vi "Serial Transmitter.vi"(9 "Robot":T1={"id"=0, "function"=enum."Attacker", "x"=0.0, "y"=0.0, "orientation"=0.0, "v_tangent"=0.0, "v_normal"=0.0, "v_ang"=0.0, "kick_x"=0.0, "kick_z"=0.0, "dribble"=FALSE, "Timestamp"=timestamp(0 s since 1904-01-01), "estimatives"={"est_v_tangent"=0.0, "est_v_normal"=0.0, "est_vx"=0.0, "est_vy"=0.0, "Pos Robot Est"=[]}, "dest_x_kick"=0.0, "dest_y_kick"=0.0, "Gap Coord"=[], "States"=enum."GoToTangent", "Path "=[], "Path  Smooth"=[], "Dest"=[], "vx_desired"=0.0, "vy_desired"=0.0, "slowBehavior"=FALSE, "VSSStates"=enum."Pass"}, 10 "Porta:":refnum<visa-resource-name>) -> (0 "error out":errorcluster)   [LabVIEW 2023]
uses:
  Vision_class/Old vision/Controls/AI Robot.ctl
  Vision_class/Old vision/Controls/Functions Enum.ctl
  Vision_class/Old vision/Controls/AttackerStates.ctl
  Vision_class/Old vision/Controls/PathDests.ctl
  Vision_class/Old vision/Controls/PathDest.ctl
  Game_class/Navigation/VSSNavigation/VSSAttackerStates.ctl
  <vilib>/Instr/_visa.llb/VISA Configure Serial Port (Instr).vi
panel:
  out "Array":u8[](array[numeric]) format="%02x"
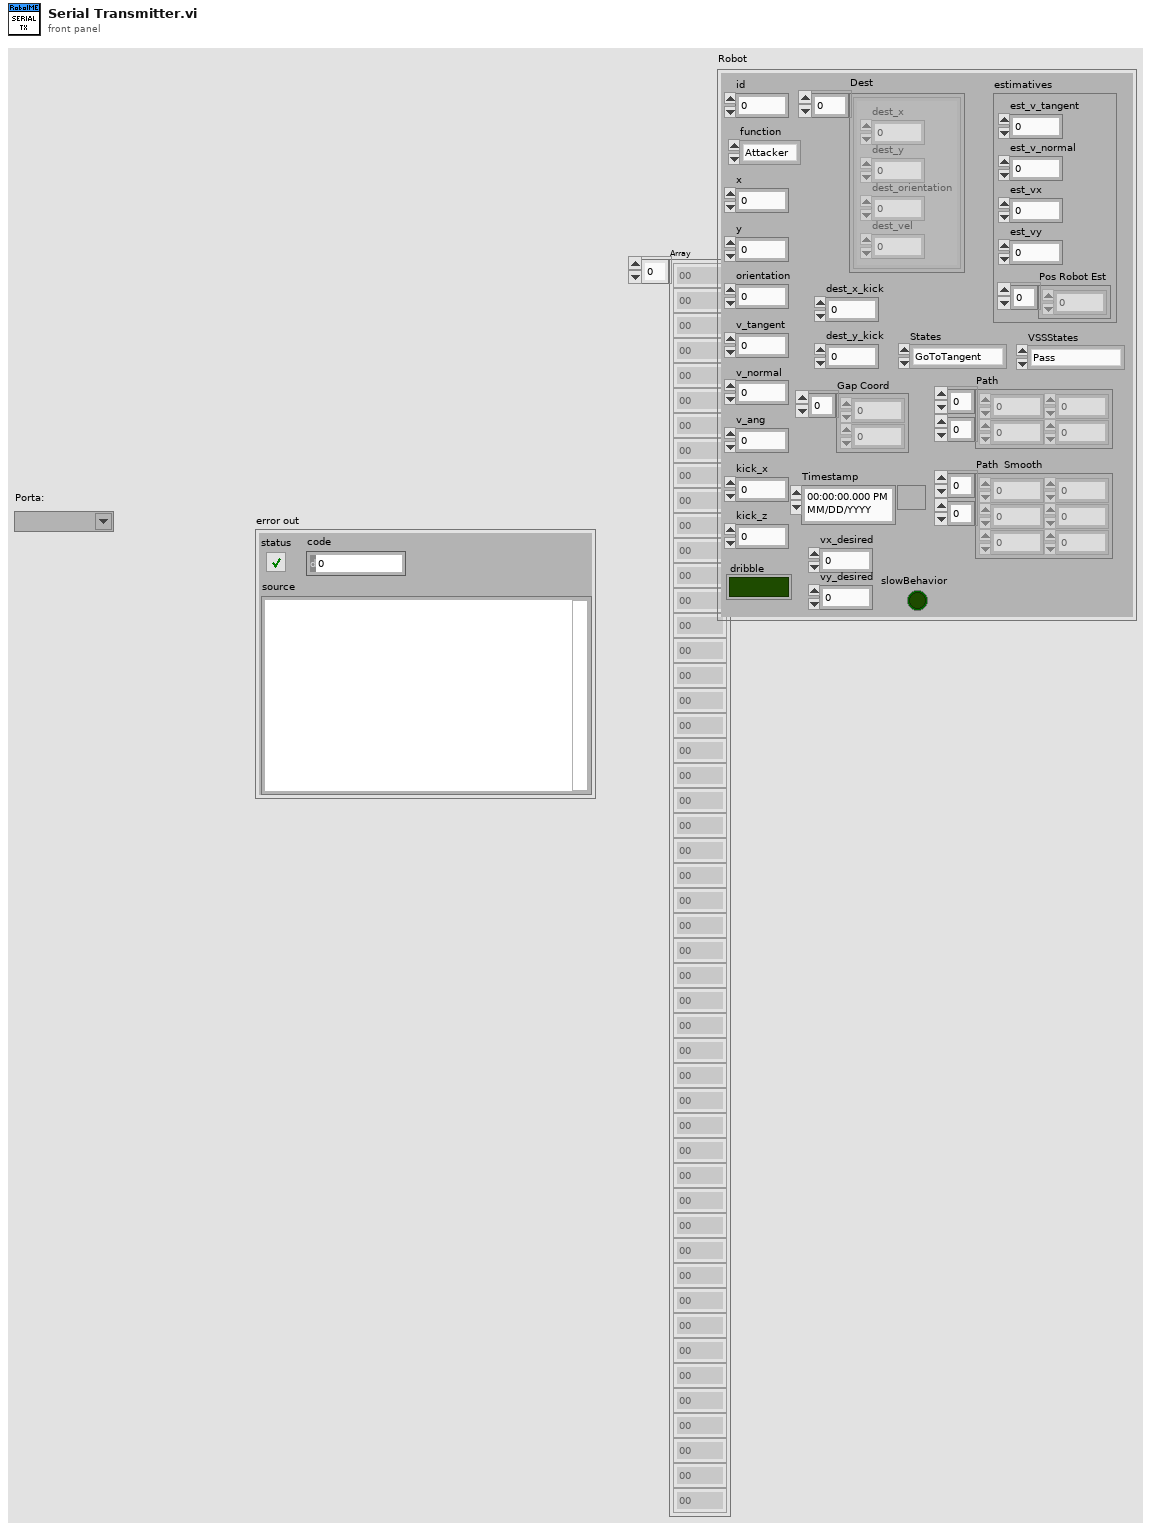
[diagram p1: front panel]
types:
  T1 = typedef "AI Robot.ctl" = cluster{"id":u32, "function":T2, "x":dbl, "y":dbl, "orientation":dbl, "v_tangent":dbl, "v_normal":dbl, "v_ang":dbl, "kick_x":dbl, "kick_z":dbl, "dribble":bool, "Timestamp":timestamp, "estimatives":cluster{"est_v_tangent":dbl, "est_v_normal":dbl, "est_vx":dbl, "est_vy":dbl, "Pos Robot Est":dbl[]}, "dest_x_kick":dbl, "dest_y_kick":dbl, "Gap Coord":dbl[], "States":T3, "Path ":dbl[][], "Path  Smooth":dbl[][], "Dest":T4, "vx_desired":dbl, "vy_desired":dbl, "slowBehavior":bool, "VSSStates":T6}
  T2 = typedef "Functions Enum.ctl" = enum16{"2nd Striker", "Attacker", "Goalie", "Defender", "Striker", "Goto 0", "Dummy", "Kicker", "ZigZag 0", "ZigZag 1", "ZigZag 2", "ZigZag 3", "ZigZag 4", "ZigZag 5", "ZigZag 6", "ZigZag 7", "ZigZag 8", ""}
  T3 = typedef "AttackerStates.ctl" = enum16{"Pass", "GoToTangent", "BallGetting", "GoToKick", ""}
  T4 = typedef "PathDests.ctl" = T5[]
  T5 = typedef "PathDest.ctl" = cluster{"dest_x":dbl, "dest_y":dbl, "dest_orientation":dbl, "dest_vel":dbl}
  T6 = typedef "VSSAttackerStates.ctl" = enum16{"Pass", "GoToTangent", "BallGetting", "GoToKick", "Rotate anti-clockwise", "Rotate Clockwise", ""}
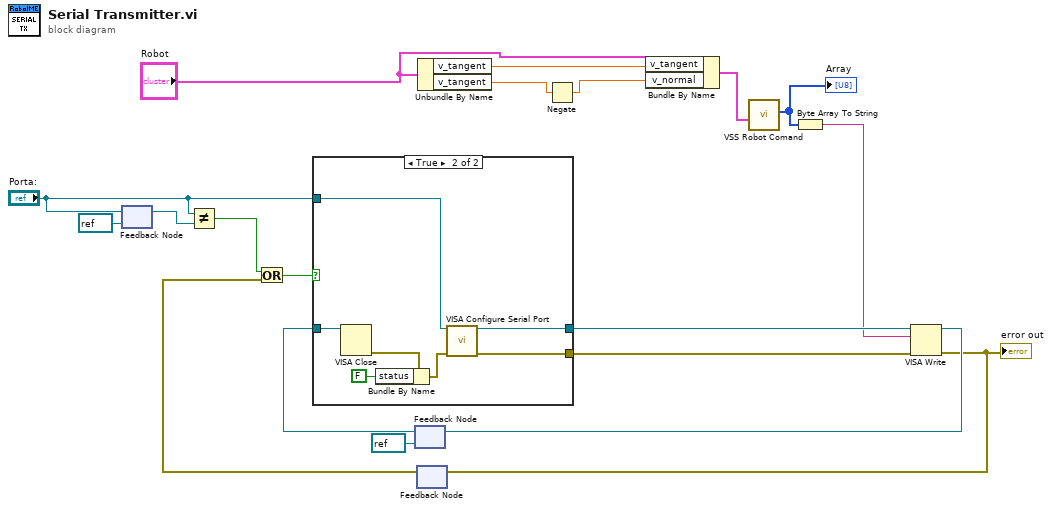
[diagram p0: block diagram]
diagram:
  n1 = feedback #1(refnum<visa-resource-name> refnum ("Porta?")) -> (w19:refnum<visa-resource-name>)
  n2 = feedback-in #1("Porta:") -> ()
  n3 = Not Equal?(x="Porta:", y=w19) -> (x != y?=w9:bool)
  n4 = feedback #2(refnum<visa-resource-name> refnum ("VISA resource name out")) -> (w18:refnum<visa-resource-name>)
  n5 = feedback #3() -> (w8:errorcluster)  [unwired: 1 in]
  n6 = Or(x=w9, y=w8) -> (x .or. y?=w10:bool)
  n7 = case shown="True" w10 {
    tunnel: [_ w25] -> w14
    tunnel: [w20 w26] -> w15
    tunnel: "Porta:" -> [_ w21]
    tunnel: w18 -> [w20 w24]
    frame False {
    }
    frame True {
      n8 = VISA Close(VISA resource name=w24) -> (error out=w23:errorcluster)  [unwired: 1 in]
      n9 = Bundle By Name(cluster=w23, "status"=FALSE) -> (w22:errorcluster)
      n10 = call-poly "VISA Configure Serial Port"("VISA resource name"=w21, "error in (no error)"=w22) -> ("VISA resource name out"=w26:refnum<visa-resource-name>, "error out"=w25:errorcluster)  [unwired: 12 in]
    }
  }
  n11 = Unbundle By Name("Robot") -> ("v_tangent"=w6:dbl, "v_tangent"=w5:dbl)
  n12 = Negate(x=w5) -> (-x=w4:dbl)
  n13 = Bundle By Name(cluster="Robot", "v_tangent"=w6, "v_normal"=w4) -> (w1:T1)
  n14 = call "VSS Robot Comand.vi"("Robot"=w1) -> ("Array"=w3:u8[])  [unwired: 10 in]
  "Array" <- w3
  n15 = Byte Array To String(unsigned byte array=w3) -> (string=w13:string)
  n16 = VISA Write(VISA resource name=w15, write buffer=w13, error in (no error)=w14) -> (VISA resource name out=w12:refnum<visa-resource-name>, error out=w11:errorcluster)  [unwired: 1 out]
  "error out" <- w11
  n17 = feedback-in #2(w12) -> ()
  n18 = feedback-in #3(w11) -> ()
